vi "toUNIX-Epoch.vi"(11 "Epoch in":refnum<class "Epoch.UTC.lvclass">) -> (2 "Unix Epoch Time":i64, 3 "Epoch":refnum<class "Epoch.UTC.lvclass">)   [LabVIEW 2013]
uses:
  Epoch.UTC.lvclass
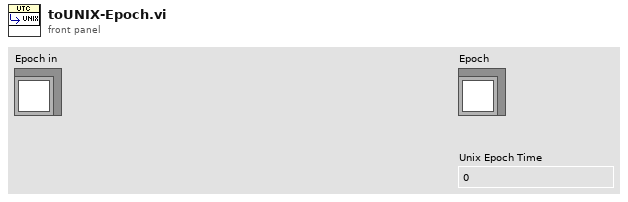
[diagram p1: front panel]
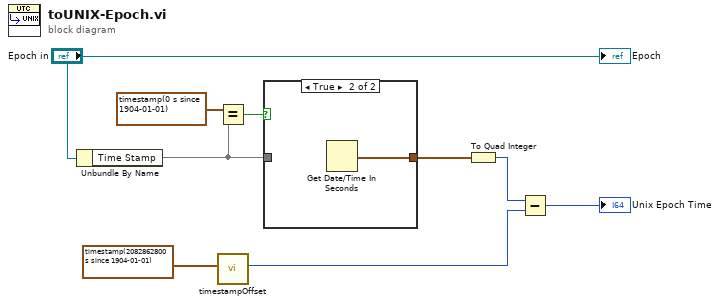
[diagram p0: block diagram]
diagram:
  n1 = Unbundle By Name("Epoch in") -> ("Time Stamp"=w7)
  n2 = Equal?(x=timestamp(0 s since 1904-01-01), y=w7) -> (x = y?=w8:bool)
  n3 = call "timestampOffset.vi"("Reference Time"=timestamp(2082862800 s since 1904-01-01) ("current time")) -> ("Timestamp Offset"=w4:i64)  [unwired: 10 in]
  n4 = case shown="True" w8 {
    tunnel: [w10 w11] -> w3
    tunnel: w7 -> [w10 _]
    frame False {
    }
    frame True {
      n5 = Get Date/Time In Seconds() -> (seconds since 1Jan1904=w11:timestamp)
    }
  }
  n6 = To Quad Integer(1:w3) -> (0:w2:i64)
  n7 = Subtract(x=w2, y=w4) -> (x-y=→"Unix Epoch Time":i64)
  "Epoch" <- "Epoch in"
